vi "Prepare_For_Close.vi"(8 "error in (no error)":errorcluster, 9 "Project path":path, 10 "use build cache":bool, 11 "AB_Source_PackedItem in":refnum<class "AB_Source_PackedItem.lvclass">) -> (0 "error out":errorcluster, 3 "AB_Source_PackedItem out":refnum<class "AB_Source_PackedItem.lvclass">)   [LabVIEW 2020, in "AB_Source_PackedItem.lvclass"]
uses:
  <vilib>/AppBuilder/AB_Classes/Source/PackedItem/AB_Source_PackedItem.lvclass
  <vilib>/AppBuilder/AB_Classes/Source/PackedItem/AB_Source_PackedItem.lvclass/AB_Source_PackedItem.ctl
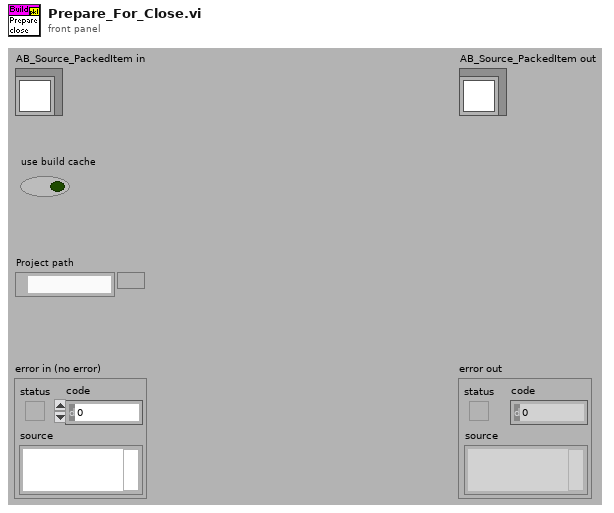
[diagram p1: front panel]
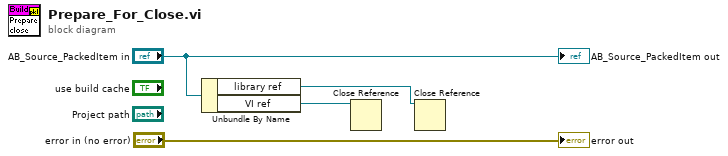
[diagram p0: block diagram]
diagram:
  n1 = Unbundle By Name("AB_Source_PackedItem in") -> ("library ref"=w2:refnum<vi>, "VI ref"=w3:refnum<vi>)
  n2 = Close Reference(reference=w3) -> ()  [unwired: 1 in, 1 out]
  n3 = Close Reference(reference=w2) -> ()  [unwired: 1 in, 1 out]
  "error out" <- "error in (no error)"
  "AB_Source_PackedItem out" <- "AB_Source_PackedItem in"
